vi "find_contours.vi"(11 "image in":T1) -> (2 "Source Image Points":cluster{"X":dbl, "Y":dbl}[](array[cluster]), 3 "image out":T1)   [LabVIEW 2017]
uses:
  <vilib>/vision/Image Controls.llb/IMAQ Image.ctl
  <vilib>/vision/Contour.llb/IMAQ Contour Curve Extraction.ctl
  <vilib>/vision/Contour.llb/IMAQ Connect Range Setting.ctl
  <vilib>/vision/NI_Vision_Development_Module.lvlib
panel:
  out "display image 1":T1(plugin-control)
  out "display image 2":T1(plugin-control)
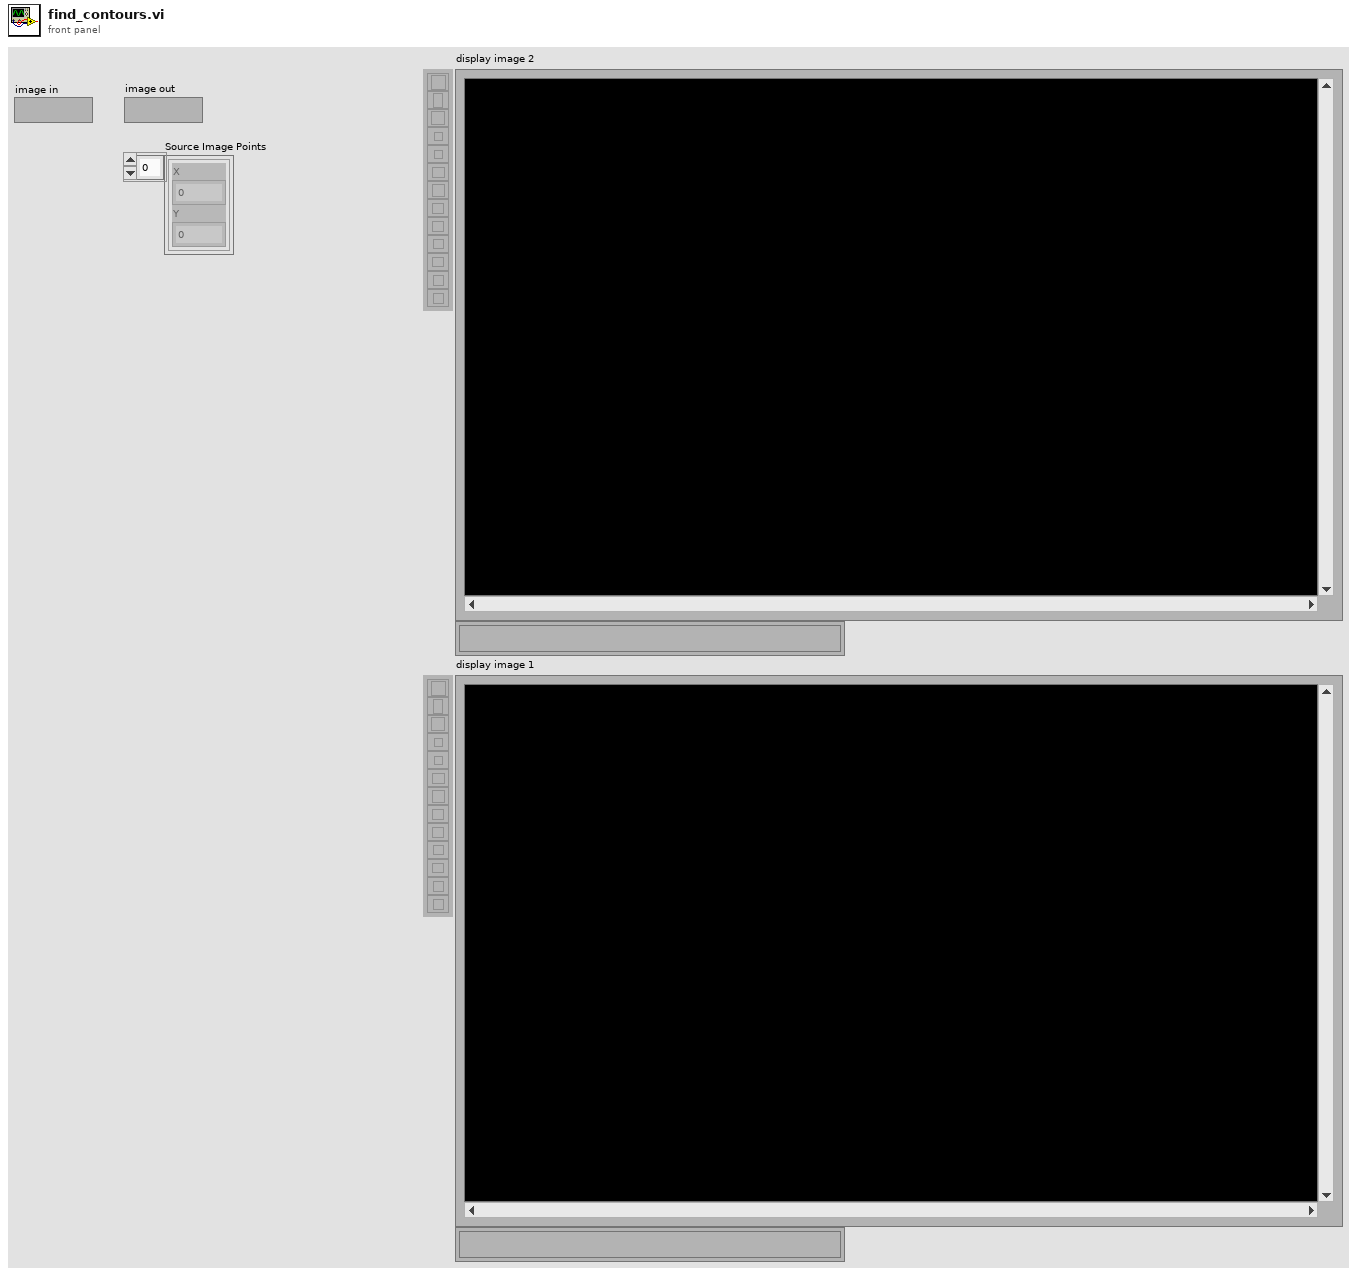
[diagram p1: front panel]
types:
  T1 = typedef "IMAQ Image.ctl" = refnum<image>
  T2 = cluster{"Overlay?":bool, "Color":u32, "Width":u32, "Maintain Width?":bool}
  T3 = enum16{"Rect Left To Right", "Rect Right To Left", "Rect Top To Bottom", "Rect Bottom To Top", "Annulus Inner To Outer", "Annulus Outer To Inner", "Annulus Start Angle To End Angle", "Annulus End Angle To Start Angle"}
  T4 = typedef "IMAQ Connect Range Setting.ctl" = cluster{"Match Constraints":u32, "Min":dbl, "Max":dbl}
  T5 = cluster{"Global Rectangle":i32[], "Contours":cluster{"ID":enum32{"External", "Internal"}, "Type":u32, "Coordinates":i32[]}[]}
  T6 = typedef "IMAQ Contour Curve Extraction.ctl" = cluster{"Extraction Mode":u32, "Edge Threshold":i32, "Edge Filter Size":u32, "Min Length":i32, "Search Step Size":i32, "Max Endpoint Gap":i32, "Subpixel":bool}
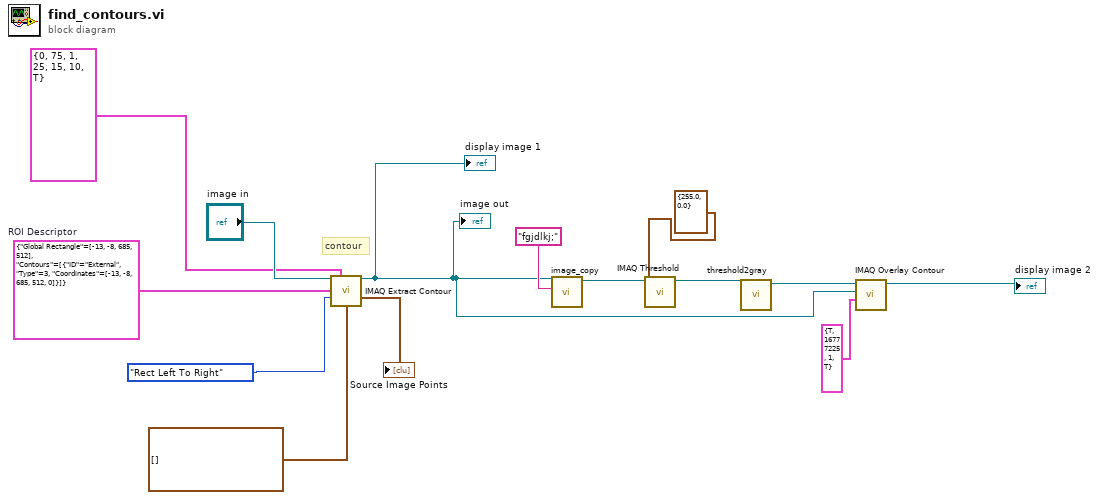
[diagram p0: block diagram]
diagram:
  w11 = T5 {"Global Rectangle"=[-13, -8, 685, 512], "Contours"=[{"ID"=enum."External", "Type"=3, "Coordinates"=[-13, -8, 685, 512, 0]}]}  # ROI Descriptor
  # "contour"
  n1 = call "IMAQ Extract Contour"("Source Image"="image in", "Curve Extraction"=T6 {"Extraction Mode"=0, "Edge Threshold"=75, "Edge Filter Size"=1, "Min Length"=25, "Search Step Size"=15, "Max Endpoint Gap"=10, "Subpixel"=TRUE}, "ROI Descriptor"=w11, "Search Direction"=T3."Rect Left To Right", "Curve Connection"=T4[] []) -> ("Source Image Out"=w1:T1, "Source Image Points"=→"Source Image Points":cluster{"X":dbl, "Y":dbl}[])  [unwired: 3 in, 6 out]
  "image out" <- w1
  "display image 1" <- w1
  n2 = call "image_copy.vi"("buffer name"="fgjdlkj;" ("Image Name"), "image in"=w1) -> ("imgae out"=w3:T1)  [unwired: 9 in]
  n3 = call "IMAQ Threshold"("Range"=cluster{"Lower value":sgl, "Upper value":sgl} {"Lower value"=255.0, "Upper value"=0.0}, "Image Src"=w3) -> ("Image Dst Out"=w6:T1)  [unwired: 4 in, 5 out]
  n4 = call "threshold2gray.vi"("threshold image"=w6) -> ("grayscale image"=w5:T1)  [unwired: 10 in]
  n5 = call "IMAQ Overlay Contour"("Contour Points Settings"=T2 {"Overlay?"=TRUE, "Color"=16777225, "Width"=1, "Maintain Width?"=TRUE}, "Contour Image"=w1, "Image"=w5) -> ("Image Out"=→"display image 2":T1)  [unwired: 3 in, 5 out]
